vi "Untitled 4.vi"() -> ()   [LabVIEW 2016]
uses:
  Tarea_ZTN/Global 1.vi
panel:
  in  "Stop Button 1":bool
  out "Boolean":bool
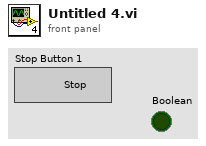
[diagram p1: front panel]
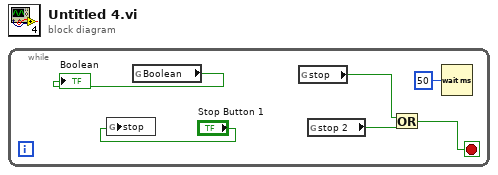
[diagram p0: block diagram]
diagram:
  n1 = while {
    stop <- w2 stop-if-true
    n2 = global write "Global 1.vi" "stop"("Stop Button 1") -> ()
    n3 = global read "Global 1.vi" "Boolean"() -> (→"Boolean":bool)
    n4 = global read "Global 1.vi" "stop"() -> (w3:bool)
    n5 = global read "Global 1.vi" "stop 2"() -> (w4:bool)
    n6 = Or(x=w3, y=w4) -> (x .or. y?=w2:bool)
    n7 = Wait (ms)(milliseconds to wait=u32 50) -> ()  [unwired: 1 out]
  }
